vi "Write Initially Open.vi"(10 "Initially Open?":bool, 11 "Flex Dialog in":refnum<class "Flex UI Dialog.lvclass">) -> (3 "Flex Dialog out":refnum<class "Flex UI Dialog.lvclass">)   [LabVIEW 2016, in "Flex UI Dialog.lvclass"]
uses:
  Flex UI Dialog.lvclass
  Flex UI Dialog.lvclass/Flex UI Dialog.ctl
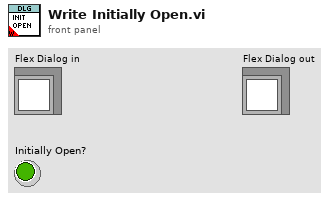
[diagram p1: front panel]
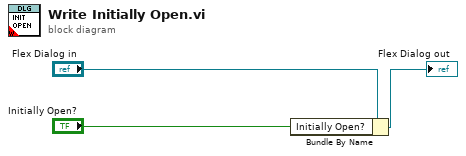
[diagram p0: block diagram]
diagram:
  n1 = Bundle By Name(cluster="Flex Dialog in", "Initially Open?"="Initially Open?") -> (→"Flex Dialog out":refnum<class "Flex UI Dialog.lvclass">)
